vi "ReversedEngineering SyncUmlFromCode.vi"(0 "SyncAction":T1, 1 "ClassPath":path, 2 "NodeRef":refnum<class "AbstractNode.lvclass">, 3 "GraphRef":refnum<class "Graph.lvclass">, 4 "IgnoreClasses":path[](array[path]), 5 "error in (no error)":errorcluster, 6 "ClassName(needed for lllbs)":string, 7 "graphics":refnum<class "Graphics.lvclass">, 8 "IterationNo":i32, 9 "grid":refnum<class "Grid.lvclass">, 10 "IterationsN":i32) -> (13 "Cancelled":bool, 14 "ClassName":string, 15 "attributes":string, 16 "methods":string, 18 "ClassesEvaluated":path[](array[path]), 19 "error out":errorcluster)   [LabVIEW 2020]
uses:
  <resource>/Framework/Providers/Open_GDS/UML/ReversedEngineering/private/ReversedEngineering SyncUmlFromCodeActions.ctl
  <resource>/Framework/Providers/Open_GDS/UML/AbstractNode_class/AbstractNode.lvclass
  <resource>/Framework/Providers/Open_GDS/UML/Graph_class/Graph.lvclass
  <resource>/Framework/Providers/Open_GDS/UML/Graphics_class/Graphics.lvclass
  <resource>/Framework/Providers/Open_GDS/UML/Grid_class/Grid.lvclass
  <resource>/Framework/Providers/Open_GDS/UML/ReversedEngineering/ReversedEngineering ClassInfoType.ctl
  <resource>/Framework/Providers/Open_GDS/UML/UMLEditor/UMLEditor_VisibilityType.ctl
  <resource>/Framework/Providers/Open_GDS/UML/ReversedEngineering/ReversedEngineering AttributeInfoType.ctl
  <resource>/Framework/Providers/Open_GDS/ClassProviders/Common/CommonVIs/CommonVIs_AttributeDataType.ctl
  <resource>/Framework/Providers/Open_GDS/UML/ReversedEngineering/ReversedEngineering_ClassDependencyDetailsType.ctl
  <resource>/Framework/Providers/Open_GDS/ClassProviders/Common/ScriptingFunctions/SubVIs/Scripting_ViDependencyType.ctl
  <resource>/Framework/Providers/Open_GDS/UML/UMLEditor/UMLEditor BusyDialogAction.ctl
  <resource>/Framework/Providers/Open_GDS/UML/ReversedEngineering/ReversedEngineering RecursiveSearchElements.ctl
  <resource>/Framework/Providers/Open_GDS/UML/AbstractEdge_class/AbstractEdge.lvclass
  <resource>/Framework/Providers/Open_GDS/UML/UmlEditor_class/UmlEditor.lvclass
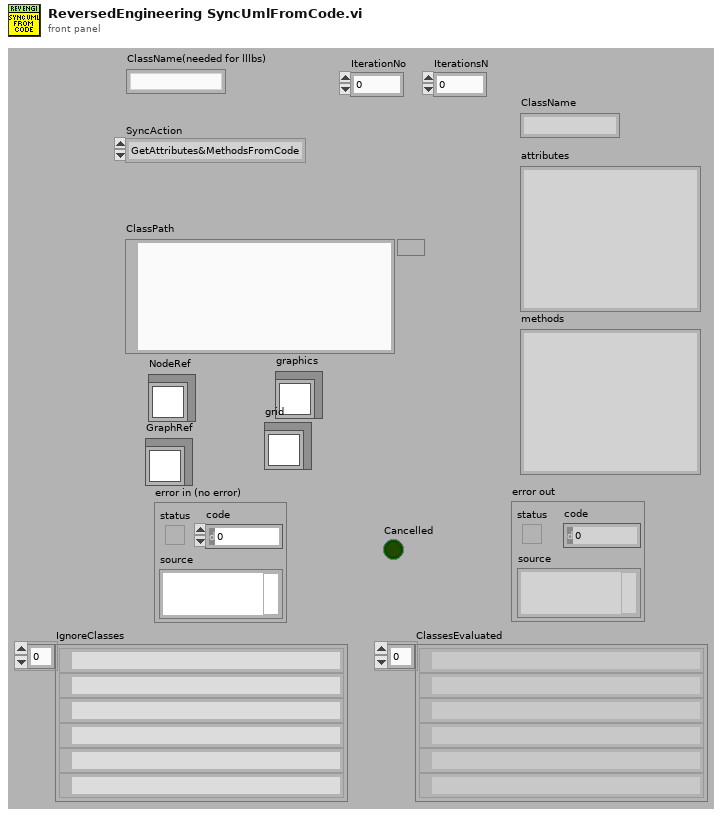
[diagram p1: front panel]
types:
  T1 = typedef "ReversedEngineering SyncUmlFromCodeActions.ctl" = enum16{"GetAttributes&MethodsFromCode", "GetAll"}
  T2 = typedef "ReversedEngineering ClassInfoType.ctl" = cluster{"classPath":path, "inherits":bool, "baseClasses":path[], "compAggClasses":path[], "noOfCompObj":i32[], "aggClasses":path[], "noOfAgg":i32[], "depClasses":path[], "methods":string[], "methodPuplic":T3[], "objectAttrib":T4[], "classAttrib":T4[], "ClassDesc":string, "DependencyDetails":T6[], "Interface":bool, "ParentInterfaces":path[]}
  T3 = typedef "UMLEditor_VisibilityType.ctl" = enum16{"Public", "Private", "Protected"}
  T4 = typedef "ReversedEngineering AttributeInfoType.ctl" = cluster{"name":string, "type":T5, "dimension":i32, "typeName":string, "typePath":path, "visibility":T3}
  T5 = typedef "CommonVIs_AttributeDataType.ctl" = enum16{"UINT8", "INT8", "UINT16", "INT16", "UINT32", "INT32", "UINT64", "INT64", "SGL", "DBL", "EXT", "CSG", "CDB", "CXT", "TimeStamp", "STRING", "PATH", "BOOL", "ENUM", "RefNum", "VIRefNum", "LabVIEW Class", "Cluster", "Variant", "TypeDef", "Waveform", "LabVIEW Object", "Other", "void"}
  T6 = typedef "ReversedEngineering_ClassDependencyDetailsType.ctl" = cluster{"DepClassPath":path, "ThisVIs/Ctls":path[], "Dependent_VIs/Ctls":path[], "ViDependecyType":T7[]}
  T7 = typedef "Scripting_ViDependencyType.ctl" = enum16{"N/A", "Launches"}
  T8 = typedef "ReversedEngineering RecursiveSearchElements.ctl" = enum16{"TopVi", "Class", "Dir", "Dir(rec.)"}
  T9 = typedef "UMLEditor BusyDialogAction.ctl" = enum16{"Initialize", "Open(VIs)", "Open(i)", "Send_I-Value", "SendStatusMessage", "GetBusyDialogStatus", "Close", "Quit"}
  T10 = typedef "UMLEditor_SyncOptions.ctl" = cluster{"IgnoreInstrLib":bool, "IgnoreUserLib":bool, "IgnoreViLib":bool}
  T11 = typedef "ReversedEngineering TypeDefType.ctl" = cluster{"TypeDefName":string, "TypeDefPath":path, "TypeDefAttribInfo":T4[]}
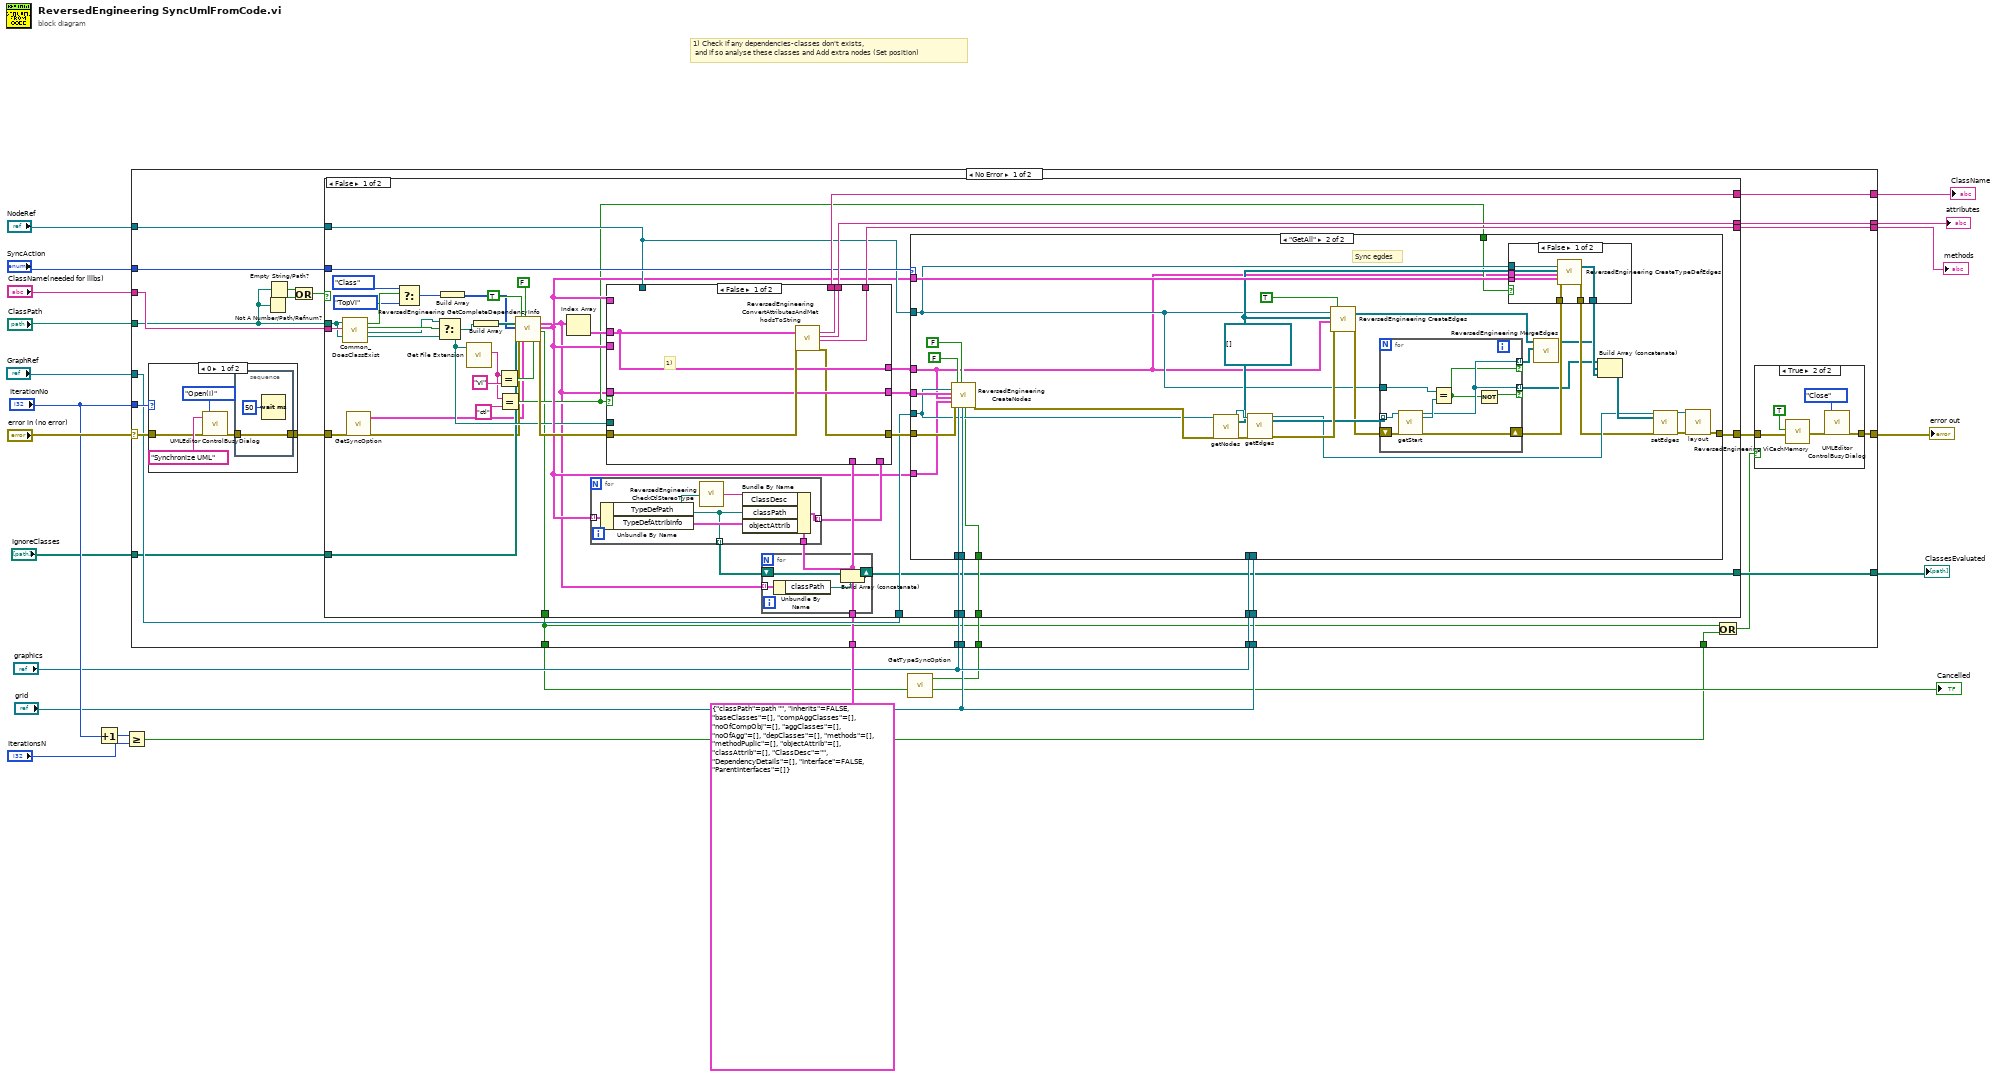
[diagram p0: block diagram]
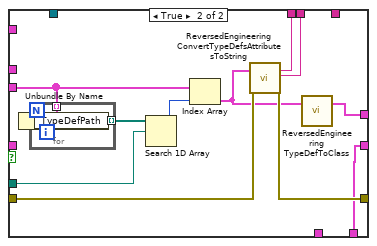
[diagram p4: hidden frame]
diagram:
  # "1) Check if any dependencies-classes don't exists,\n and if so analyse these classes and Add extra nodes (Set position)"
  n1 = Increment(x="IterationNo") -> (x+1=w10:i32)
  n2 = Greater Or Equal?(x=w10, y="IterationsN") -> (x >= y?=w1:bool)
  n3 = call <resource>:"GetTypeSyncOption.vi"() -> ("TypeSyncOption"=w5:bool)  [unwired: 1 in, 18 out]
  n4 = case shown="No Error" "error in (no error)" {
    selector: "error in (no error)" -> [w44 w189]
    tunnel: [w42 w189] -> w20
    tunnel: "ClassPath" -> [w28 _]
    tunnel: [w48 _] -> w19
    tunnel: [w47 _] -> w18
    tunnel: [w46 _] -> w16
    tunnel: "SyncAction" -> [w40 _]
    tunnel: "NodeRef" -> [w39 _]
    tunnel: "GraphRef" -> [w37 _]
    tunnel: "ClassName(needed for lllbs)" -> [w45 _]
    tunnel: "IterationNo" -> [w41 _]
    tunnel: T2 {"classPath"=path "", "inherits"=FALSE, "baseClasses"=[], "compAggClasses"=[], "noOfCompObj"=[], "aggClasses"=[], "noOfAgg"=[], "depClasses"=[], "methods"=[], "methodPuplic"=[], "objectAttrib"=[], "classAttrib"=[], "ClassDesc"="", "DependencyDetails"=[], "Interface"=FALSE, "ParentInterfaces"=[]} ("classInfo") -> [w31 _]
    tunnel: "graphics" -> [w36 _]
    tunnel: "grid" -> [w35 _]
    tunnel: "graphics" -> [w34 _]
    tunnel: "grid" -> [w33 _]
    tunnel: w5 -> [w32 _]
    tunnel: "IgnoreClasses" -> [w30 _]
    tunnel: [w29 _] -> w3
    tunnel: [w23 _] -> w2
    tunnel: w1 -> [w24 _]
    frame No Error {
      n5 = case shown="0" w41 {
        tunnel: w44 -> [w182 w188]
        tunnel: [w181 w188] -> w43
        frame 0 {
          n6 = call <resource>:"UMLEditor ControlBusyDialog.vi"("Title/StatusText"="Synchronize UML", "error in (no error)"=w182, "Action(SendStatusMessage)"=UMLEditor_BusyDialogAction."Open(i)" ("Action")) -> ("error out"=w185:errorcluster)  [unwired: 1 in, 15 out]
          n7 = stacked-sequence {
            tunnel: [w187] -> w181
            tunnel: w185 -> [w187]
            frame #0 {
              n8 = Wait (ms)(milliseconds to wait=u32 50) -> ()  [unwired: 1 out]
            }
          }
        }
        frame Default {
        }
      }
      n9 = Not A Number/Path/Refnum?(number/path/refnum=w28) -> (NaN/Path/Refnum?=w26:bool)
      n10 = Empty String/Path?(string/path=w28) -> (empty?=w27:bool)
      n11 = Or(x=w27, y=w26) -> (x .or. y?=w25:bool)
      n12 = case shown="False" w25 {
        tunnel: [w91 _] -> w48
        tunnel: [w90 _] -> w47
        tunnel: [w88 _] -> w46
        tunnel: w45 -> [w86 _]
        tunnel: w43 -> [w52 w174]
        tunnel: w40 -> [w83 _]
        tunnel: w39 -> [w82 _]
        tunnel: [w78 w174] -> w38
        tunnel: w37 -> [w77 _]
        tunnel: w36 -> [w76 _]
        tunnel: w35 -> [w75 _]
        tunnel: w34 -> [w69 _]
        tunnel: w33 -> [w68 _]
        tunnel: w32 -> [w67 _]
        tunnel: w31 -> [w66 _]
        tunnel: w30 -> [w57 _]
        tunnel: [w54 _] -> w29
        tunnel: w28 -> [w53 _]
        tunnel: [w49 _] -> w23
        frame False {
          n13 = call <resource>:"Common_DoesClassExist.vi"("ClassPath"=w53, "ClassName"=w86) -> ("ClassExists"=w74:bool, "llb-class"=w85:bool, "llb/LvCLass-Path"=w84:path)  [unwired: 15 out]
          n14 = call <resource>:"GetSyncOption.vi"("error in (no error)"=w52) -> ("SyncOption"=w50:T10, "error out"=w51:errorcluster)  [unwired: 16 in, 1 out]
          n15 = Select(t=ReversedEngineering_RecursiveSearchElements."Class" ("Enum"), s=w74, f=ReversedEngineering_RecursiveSearchElements."TopVi" ("Enum")) -> (s? t:f=w71:T8)
          n16 = Select(t=w84, s=w85, f=w53) -> (s? t:f=w58:path)
          n17 = Build Array(w71) -> (w70:T8[])
          n18 = call <vilib>:"Get File Extension.vi"("file"=w58) -> ("lowercase file extension"=w61:string)  [unwired: 1 in, 9 out]
          n19 = Build Array(w58) -> (w94:path[])
          n20 = Equal?(x=w61, y="vi") -> (x = y?=w62:bool)
          n21 = Equal?(x=w61, y="ctl" ("regular expression")) -> (x = y?=w59:bool)
          n22 = call <resource>:"ReversedEngineering GetCompleteDependencyInfo.vi"("path"=w94, "SearchElements"=w70, "IgnoreClasses"=w57, "error in (no error)"=w51, "Only Create this class and its dependencis"=TRUE, "SyncOption"=w50, "Only analyse this class methods and attributes(False)"=FALSE ("Only analyse this clas methods and attributes(False)"), "CreateApplicationNode"=w62) -> ("classInfos"=w56:T2[], "TypeDefs"=w64:T11[], "Cancelled"=w49:bool, "error out"=w92:errorcluster)  [unwired: 8 out]
          n23 = Index Array(array=w56) -> (element=w89:T2)  [unwired: 1 in]
          n24 = for {
            tunnel: w64 -> [w103] mode=indexing
            tunnel: w66 -> [w104]
            tunnel: [w101] -> w65 mode=indexing
            tunnel: [w99] -> w55 mode=indexing
            n25 = Unbundle By Name(w103) -> ("TypeDefPath"=w99:path, "TypeDefAttribInfo"=w102:T4[])
            n26 = call <resource>:"ReversedEngineering CheckCtlStereoType.vi"("TypeDefPath"=w99) -> ("ClassDesc"=w100:string)
            n27 = Bundle By Name(cluster=w104, "ClassDesc"=w100, "classPath"=w99, "objectAttrib"=w102) -> (w101:T2)
          }
          n28 = case shown="False" w59 {
            tunnel: w92 -> [w160 w169]
            tunnel: [w159 w171] -> w91
            tunnel: [w158 _] -> w90
            tunnel: w89 -> [w156 _]
            tunnel: [w157 w170] -> w88
            tunnel: [w154 w168] -> w79
            tunnel: w56 -> [w155 _]
            tunnel: w82 -> [_ _]
            tunnel: w64 -> [_ _]
            tunnel: [w156 w167] -> w81
            tunnel: [w155 w166] -> w80
            tunnel: w66 -> [_ _]
            tunnel: w65 -> [_ w166]
            tunnel: w64 -> [_ w164]
            tunnel: w58 -> [_ w162]
            frame False {
              # "1)"
              n29 = call <resource>:"ReversedEngineering ConvertAttributesAndMethodsToString.vi"("classInfo"=w156, "error in (no error)"=w160) -> ("className"=w157:string, "attributes"=w159:string, "methods"=w158:string, "error out"=w154:errorcluster)  [unwired: 14 out]
            }
            frame True {
              n30 = for {
                tunnel: w164 -> [w173] mode=indexing
                tunnel: [w172] -> w163 mode=indexing
                n31 = Unbundle By Name(w173) -> ("TypeDefPath"=w172:path)
              }
              n32 = Search 1D Array(1D array=w163, element=w162) -> (index of element=w161:i32)  [unwired: 1 out]
              n33 = Index Array(array=w164, index=w161) -> (element=w165:T11)
              n34 = call <resource>:"ReversedEngineering ConvertTypeDefsAttributesToString.vi"("TypeDef"=w165, "error in (no error)"=w169) -> ("className"=w170:string, "attributes"=w171:string, "error out"=w168:errorcluster)  [unwired: 15 out]
              n35 = call <resource>:"ReversedEngineering TypeDefToClass.vi"("TypeDef"=w165) -> ("NodeClassInfo"=w167:T2)  [unwired: 18 out]
            }
          }
          n36 = for {
            tunnel: w56 -> [w98] mode=indexing
            shift-right: [w95] -> w54
            shift-left: w55 -> [w97]
            n37 = Unbundle By Name(w98) -> ("classPath"=w96:path)
            n38 = Build Array (concatenate)(w97, w96) -> (w95:path[])
          }
          n39 = case shown="\"GetAll\"" w83 {
            tunnel: w79 -> [w105 w122]
            tunnel: [w105 w129] -> w78
            tunnel: w82 -> [_ w116]
            tunnel: w77 -> [_ w113]
            tunnel: w81 -> [_ w110]
            tunnel: w64 -> [_ w124]
            tunnel: w80 -> [_ w119]
            tunnel: w76 -> [_ w118]
            tunnel: w75 -> [_ w117]
            tunnel: w59 -> [_ w115]
            tunnel: w69 -> [_ _]
            tunnel: w68 -> [_ _]
            tunnel: w67 -> [_ w112]
            tunnel: w64 -> [_ w111]
            frame "GetAttributes&MethodsFromCode", Default {
            }
            frame "GetAll" {
              (unwired) refnum<class "AbstractEdge.lvclass">[] []
              # "Sync egdes"
              n40 = call <resource>:"ReversedEngineering CreateNodes.vi"("GraphRefToAddNodesTo"=w113, "NodeClassInfoArray"=w119, "NodeClassInfo"=w110, "TypeDefs"=w111, "error in (no error)"=w122, "Show Methods"=FALSE, "graphics"=w118, "Show Attributes"=FALSE, "grid"=w117, "CreateTypeDefs"=w112) -> ("error out"=w114:errorcluster)  [unwired: 1 in, 8 out]
              n41 = call-dynamic "getNodes.vi"("reference"=w113, "error in (no error)"=w114) -> ("reference out"=w137:refnum<class "Graph.lvclass">, "nodes"=w123:refnum<class "AbstractNode.lvclass">[], "error out"=w136:errorcluster)  [unwired: 15 in]
              n42 = call-dynamic "getEdges.vi"("reference"=w137, "error in (no error)"=w136) -> ("reference out"=w132:refnum<class "Graph.lvclass">, "edges"=w134:refnum<class "AbstractEdge.lvclass">[], "error out"=w135:errorcluster)  [unwired: 15 in]
              n43 = call <resource>:"ReversedEngineering CreateEdges.vi"("NodeRef"=w116, "AllNodes"=w123, "NodeClassInfo"=w110, "error in (no error)"=w135, "Show Multiplicity"=TRUE) -> ("EdgesCreated"=w107:refnum<class "AbstractEdge.lvclass">[], "error out"=w127:errorcluster)  [unwired: 13 out]
              n44 = for {
                shift-right: [w149] -> _
                shift-left: w127 -> [w153]
                tunnel: w134 -> [w152] mode=indexing
                tunnel: w116 -> [w150]
                tunnel: [w148] -> w108 mode=indexing if=w147
                tunnel: [w148] -> w109 mode=indexing if=w146
                n45 = call-dynamic "getStart.vi"("reference"=w152, "error in (no error)"=w153) -> ("reference out"=w148:refnum<class "AbstractEdge.lvclass">, "startNode"=w151:refnum<class "AbstractNode.lvclass">, "error out"=w149:errorcluster)  [unwired: 14 in, 1 out]
                n46 = Equal?(x=w150, y=w151) -> (x = y?=w147:bool)
                n47 = Not(x=w147) -> (.not. x?=w146:bool)
              }
              n48 = case shown="False" w115 {
                tunnel: [w144 _] -> w128
                tunnel: w127 -> [w143 w145]
                tunnel: [w142 w145] -> w126
                tunnel: w124 -> [w141 _]
                tunnel: w123 -> [w140 _]
                tunnel: w116 -> [w139 _]
                tunnel: w110 -> [w138 _]
                frame False {
                  n49 = call <resource>:"ReversedEngineering CreateTypeDefEdges.vi"("NodeRef"=w139, "AllNodes"=w140, "NodeClassInfo"=w138, "TypeDefs"=w141, "error in (no error)"=w143) -> ("EdgesCreated"=w144:refnum<class "AbstractEdge.lvclass">[], "error out"=w142:errorcluster)  [unwired: 1 in, 12 out]
                }
                frame True {
                }
              }
              n50 = call <resource>:"ReversedEngineering MergeEdges.vi"("ExistingEdges"=w108, "EdgesCreated"=w107) -> ("EdgesOut"=w106:refnum<class "AbstractEdge.lvclass">[])  [unwired: 9 in]
              n51 = Build Array (concatenate)(w109, w106, w128) -> (w133:refnum<class "AbstractEdge.lvclass">[])
              n52 = call-dynamic "setEdges.vi"("reference"=w132, "edges"=w133, "error in (no error)"=w126) -> ("reference out"=w131:refnum<class "Graph.lvclass">, "error out"=w130:errorcluster)  [unwired: 15 in]
              n53 = call-dynamic "layout.vi"("reference"=w131, "error in (no error)"=w130) -> ("error out"=w129:errorcluster)  [unwired: 16 in, 1 out]
            }
          }
        }
        frame True {
        }
      }
      n54 = Or(x=w23, y=w24) -> (x .or. y?=w22:bool)
      n55 = case shown="True" w22 {
        tunnel: w38 -> [w175 w177]
        tunnel: [w175 w176] -> w42
        frame False {
        }
        frame True {
          n56 = call <resource>:"ReversedEngineering ViCachMemory.vi"("RemoveAllCachedViRefs(False)"=TRUE, "error in (no error)"=w177) -> ("error out"=w179:errorcluster)  [unwired: 2 in, 15 out]
          n57 = call <resource>:"UMLEditor ControlBusyDialog.vi"("error in (no error)"=w179, "Action(SendStatusMessage)"=UMLEditor_BusyDialogAction."Close") -> ("error out"=w176:errorcluster)  [unwired: 2 in, 15 out]
        }
      }
    }
    frame Error {
    }
  }
  "error out" <- w20
  "attributes" <- w19
  "methods" <- w18
  "ClassName" <- w16
  "ClassesEvaluated" <- w3
  "Cancelled" <- w2
